vi "Event Selector.vi"(8 "Error In":errorcluster, 9 "Session In":T3="cam0", 10 "Pass In Event":bool, 11 "Manual Pass In Event":T1=enum."Start Button Pressed") -> (0 "Error Out":errorcluster, 1 "Session Out":T3="cam0", 3 "Event Queue":T1[](array[typedef]))   [LabVIEW 2017]
uses:
  <vilib>/userdefined/High Color/IMAQdx.ctl
  state-manager/Event.ctl
  Sense/Camera/Colour Typedef.ctl
  <vilib>/myRIO/Instrument Drivers/Onboard IO/DIO/typedefs/DIO Reference.ctl
  <vilib>/myRIO/Common/Instrument Driver Framework/Utilities/typedefs/myRIO Generic Hardware Reference.ctl
  <vilib>/myRIO/Common/Instrument Driver Framework/Utilities/typedefs/Hardware Version Enum.ctl
  <vilib>/myRIO/Common/Instrument Driver Framework/Utilities/typedefs/myRIO v1.0 Reference.ctl
  <vilib>/myRIO/Common/Instrument Driver Framework/Utilities/typedefs/Generic FPGA Reference.ctl
  <vilib>/myRIO/Common/Instrument Driver Framework/myRIO v1.0/DIO/typedefs/DIO Channels List.ctl
  <vilib>/myRIO/Common/Instrument Driver Framework/myRIO v1.0/DIO/typedefs/DIO Channels Enum.ctl
  <vilib>/userdefined/High Color/nirio_resource_hc.ctl
  <vilib>/myRIO/Common/Instrument Driver Framework/Utilities/vis/Is FPGA Ref Available.vi
  <vilib>/myRIO/Common/Instrument Driver Framework/myRIO v1.0/DIO/vis/myRIO v1.1 Open DIO.vi
  <vilib>/myRIO/Instrument Drivers/Onboard IO/DIO/vis/Read.vi
  <vilib>/myRIO/Common/Instrument Driver Framework/Utilities/vis/Validate Channels.vi
  <vilib>/myRIO/Common/Instrument Driver Framework/myRIO v1.0/DIO/vis/myRIO v1.0 Reserve DIO.vi
  <vilib>/myRIO/Common/Instrument Driver Framework/myRIO v1.0/Resource Manager/vis/myRIO v1.0 Reserve Channel List.vi
  <vilib>/myRIO/Common/Instrument Driver Framework/myRIO v1.0/DIO/vis/myRIO v1.0 Build MUX Configuration DIO.vi
  <vilib>/myRIO/Common/Instrument Driver Framework/myRIO v1.0/Resource Manager/vis/myRIO v1.0 Reserve Channel.vi
  <vilib>/myRIO/Common/Instrument Driver Framework/myRIO v1.0/Resource Manager/vis/myRIO v1.0 Unreserve Channel.vi
  <vilib>/myRIO/Common/Instrument Driver Framework/myRIO v1.0/Resource Manager/vis/myRIO v1.0 Create Configuration List.vi
  <vilib>/myRIO/Common/Instrument Driver Framework/myRIO v1.0/Resource Manager/vis/myRIO v1.0 Build Mutex Name.vi
  Globals/Pose.vi
  <vilib>/Utility/VariantDataType/GetNumericInfo.vi
  <vilib>/Utility/error.llb/Error Cluster From Error Code.vi
  <vilib>/myRIO/Common/Instrument Driver Framework/myRIO v1.0/myRIO v1.1 Open.vi
  <vilib>/myRIO/Common/Instrument Driver Framework/Utilities/vis/IO Manager.vi
  <vilib>/myRIO/Common/Instrument Driver Framework/Utilities/vis/Configuration Manager.vi
  <vilib>/myRIO/Common/Instrument Driver Framework/myRIO v1.0/Resource Manager/vis/myRIO v1.0 Configure IO.vi
  <vilib>/myRIO/Common/Instrument Driver Framework/myRIO v1.0/myRIO v1.0 Close.vi
  <vilib>/myRIO/Common/Instrument Driver Framework/myRIO v1.0/DIO/vis/myRIO v1.0 Read DIO.vi
  Globals/Zig Zag Global.vi
  <vilib>/myRIO/Express VI/Onboard IO/DI/DI Express VI.xnode
  <vilib>/myRIO/Instrument Drivers/Onboard IO/DIO/vis/myRIO DIO Open.xnode
  <vilib>/myRIO/Instrument Drivers/Onboard IO/DIO/DIO.lvlib
panel:
  out "Line Colour":T2=enum."Blue"
  out "Line Color Confidence (0-100)":dbl=0.4775520833333333
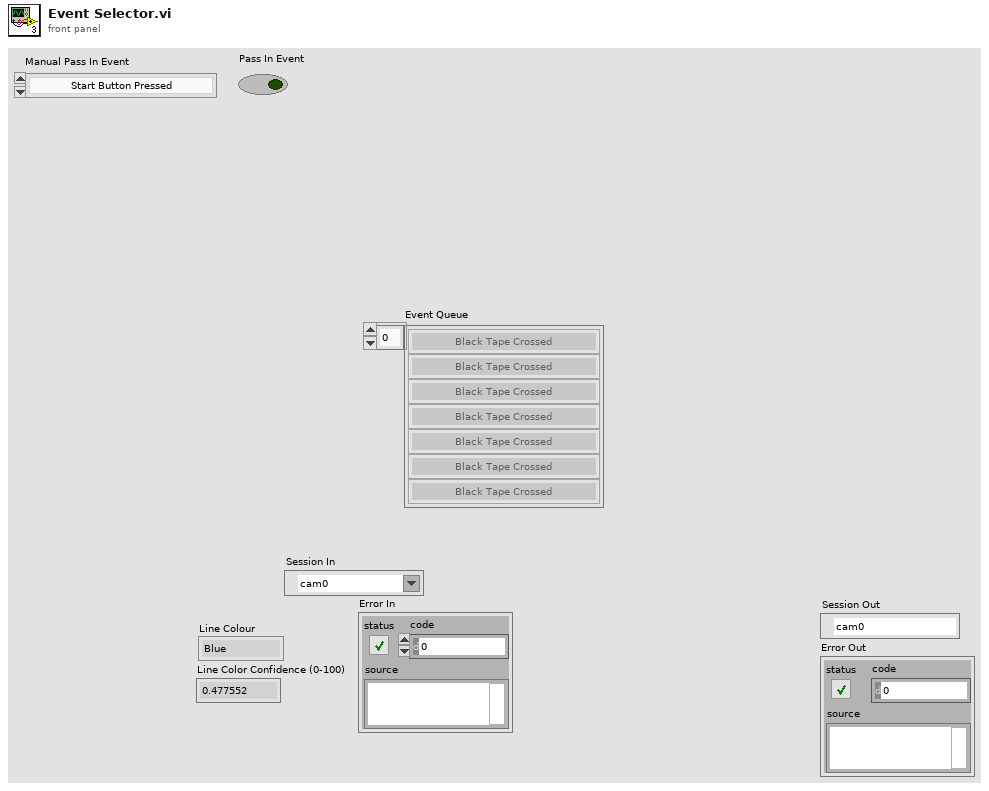
[diagram p1: front panel]
types:
  T1 = typedef "Event.ctl" = enum16{"None", "Zig Zag Finished", "Start Obstacle Avoidance", "Start Button Pressed", "Black & Yellow Tape Touched", "Black & Yellow Tape Passed", "Green Tape Crossed", "Red Tape Touched", "Rough Terrain Touched", "Black Tape Crossed", "Tape Edge Too Close", "Wall Too Close", "Rough Terrain Passed", "Ramp Passed", "Stop Button Pressed", "Recentered", "End Zone Wait Timed Out"}
  T2 = typedef "Colour Typedef.ctl" = enum16{"Yellow", "Red", "Black", "Green", "Blue", "None", "Black&Yellow"}
  T3 = typedef "IMAQdx.ctl" = refnum<k21>
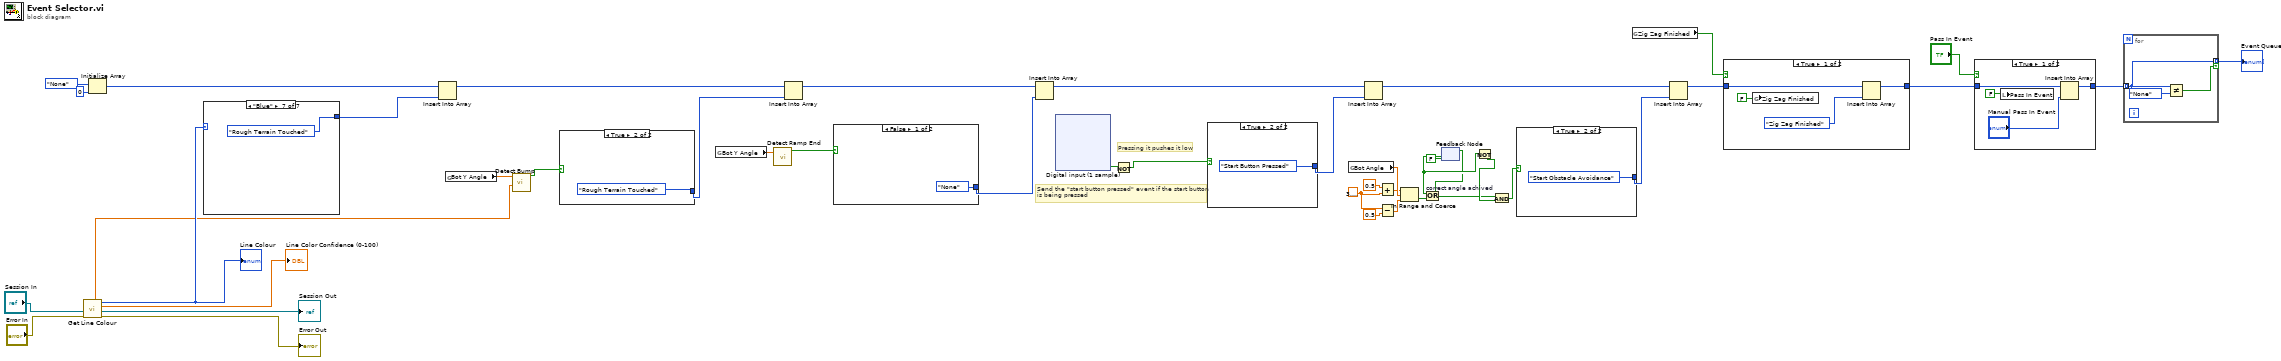
[diagram p0: block diagram]
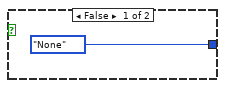
[diagram p3: hidden frame]
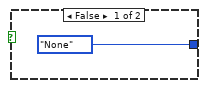
[diagram p4: hidden frame]
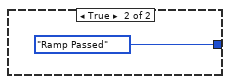
[diagram p5: hidden frame]
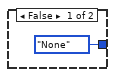
[diagram p6: hidden frame]
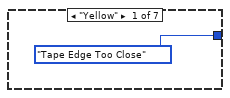
[diagram p8: hidden frame]
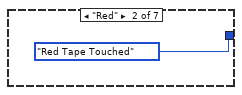
[diagram p9: hidden frame]
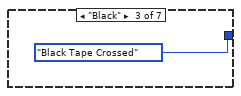
[diagram p10: hidden frame]
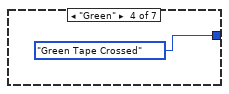
[diagram p11: hidden frame]
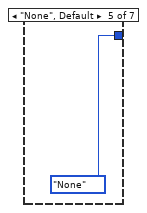
[diagram p12: hidden frame]
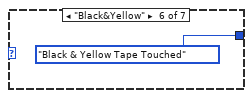
[diagram p13: hidden frame]
diagram:
  w33 = 3.141592653589793
  # "Pressing it pushes it low"
  # "Send the \"start button pressed\" event if the start button\nis being pressed"
  n1 = call "Get Line Colour.vi"("Error In"="Error In", "Session In"="Session In") -> ("Error Out"=→"Error Out":errorcluster, "Session Out"=→"Session Out":T3, "Confidence (0-100)"=→"Line Color Confidence (0-100)":dbl, "Colour"=w26:T2, "Blue"=w24:dbl)  [unwired: 5 in]
  "Line Colour" <- w26
  n2 = Initialize Array(Event."None" ("Event 2"), 0 ("dimension size")) -> (w8:T1[])
  n3 = case shown="\"Blue\"" w26 {
    tunnel: [Event."Tape Edge Too Close" ("Event 2") Event."Red Tape Touched" ("Event 2") Event."Black Tape Crossed" ("Event 2") Event."Green Tape Crossed" ("Event 2") Event."None" ("Event 2") Event."Black & Yellow Tape Touched" ("Event 2") Event."Rough Terrain Touched" ("Event 2")] -> w21
    frame "Yellow" {
    }
    frame "Red" {
    }
    frame "Black" {
    }
    frame "Green" {
    }
    frame "None", Default {
    }
    frame "Black&Yellow" {
    }
    frame "Blue" {
    }
  }
  n4 = Insert Into Array(array=w8, new element=w21) -> (w20:T1[])  [unwired: 1 in]
  n5 = global read "Pose.vi" "Bot Y Angle"() -> (w22:dbl)
  n6 = call "Detect Bump.vi"("Blue Confidence"=w24, "y angle"=w22) -> ("Bumpy Terrain"=w25:bool)  [unwired: 9 in]
  n7 = case shown="True" w25 {
    tunnel: [Event."None" ("Event 2") Event."Rough Terrain Touched" ("Event 2")] -> w19
    frame False {
    }
    frame True {
    }
  }
  n8 = global read "Pose.vi" "Bot Y Angle"() -> (w9:dbl)
  n9 = call "Detect Ramp End.vi"("y angle"=w9) -> ("Ramp Just Ended"=w23:bool)  [unwired: 10 in]
  n10 = Insert Into Array(array=w20, new element=w19) -> (w18:T1[])  [unwired: 1 in]
  n11 = case shown="False" w23 {
    tunnel: [Event."None" ("Event 2") Event."Ramp Passed" ("Event 2")] -> w17
    frame False {
    }
    frame True {
    }
  }
  n12 = Insert Into Array(array=w18, new element=w17) -> (w14:T1[])  [unwired: 1 in]
  n13 = xnode "Digital input (1 sample)"() -> ("A/DIO1 (Pin 13)"=w39:bool)  [unwired: 1 in, 1 out]
  n14 = Not(x=w39) -> (.not. x?=w16:bool)
  n15 = case shown="True" w16 {
    tunnel: [Event."None" ("Event 2") Event."Start Button Pressed" ("Event 2")] -> w13
    frame False {
    }
    frame True {
    }
  }
  n16 = global read "Pose.vi" "Bot Angle"() -> (w38:dbl)
  n17 = Insert Into Array(array=w14, new element=w13) -> (w11:T1[])  [unwired: 1 in]
  n18 = Add(x=0.5, y=w33) -> (x+y=w35:dbl)
  n19 = Subtract(x=w33, y=0.5) -> (x-y=w34:dbl)
  n20 = In Range and Coerce(upper limit=w35, x=w38, lower limit=w34) -> (In Range?=w37:bool)  [unwired: 1 out]
  n21 = feedback #1(FALSE) -> (w30:bool)
  n22 = Or "correct angle achived"(x=w30, y=w37) -> (x .or. y?=w28:bool)
  n23 = feedback-in #1(w28) -> ()
  n24 = Not(x=w30) -> (.not. x?=w29:bool)
  n25 = And(x=w28, y=w29) -> (x .and. y?=w15:bool)
  n26 = case shown="True" w15 {
    tunnel: [Event."None" ("Event 2") Event."Start Obstacle Avoidance" ("Event 2")] -> w12
    frame False {
    }
    frame True {
    }
  }
  n27 = global read "Zig Zag Global.vi" "Zig Zag Finished"() -> (w1:bool)
  n28 = Insert Into Array(array=w11, new element=w12) -> (w3:T1[])  [unwired: 1 in]
  n29 = case shown="True" w1 {
    tunnel: w3 -> [w62 w63]
    tunnel: [w61 w63] -> w2
    frame True {
      n30 = global write "Zig Zag Global.vi" "Zig Zag Finished"(FALSE ("Pass In Event")) -> ()
      n31 = Insert Into Array(array=w62, new element=Event."Zig Zag Finished" ("Event 2")) -> (w61:T1[])  [unwired: 1 in]
    }
    frame False {
    }
  }
  n32 = case shown="True" "Pass In Event" {
    tunnel: w2 -> [w66 w68]
    tunnel: [w64 w68] -> w4
    frame True {
      n33 = local write "Pass In Event"(FALSE ("Pass In Event")) -> ()
      n34 = Insert Into Array(array=w66, new element="Manual Pass In Event") -> (w64:T1[])  [unwired: 1 in]
    }
    frame False {
    }
  }
  n35 = for {
    tunnel: [w69] -> w5 mode=indexing if=w70
    tunnel: w4 -> [w69] mode=indexing
    n36 = Not Equal?(x=w69, y=Event."None") -> (x != y?=w70:bool)
  }
  "Event Queue" <- w5
